vi "Write Body.vi"(8 "error in (no error)":errorcluster, 10 "Body":string="FLATXML", 11 "Annouce Msg in":refnum<class "Annouce Msg.lvclass">) -> (0 "error out":errorcluster, 3 "Annouce Msg out":refnum<class "Annouce Msg.lvclass">)   [LabVIEW 2013, in "Receiver.lvlib" / "Annouce Msg.lvclass"]
uses:
  Annouce Msg.lvclass
  Annouce Msg.lvclass/Annouce Msg.ctl
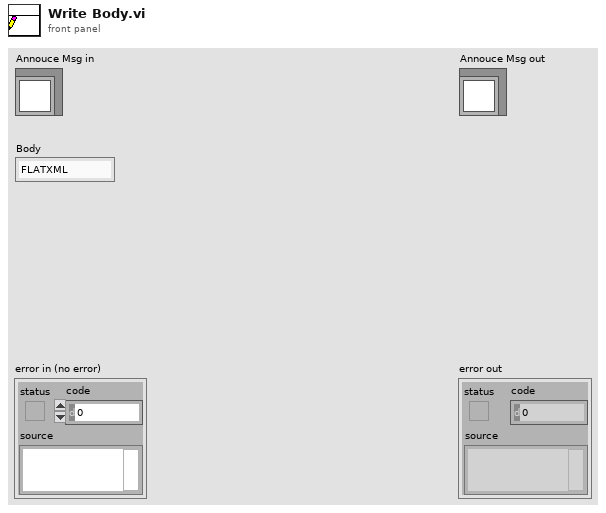
[diagram p1: front panel]
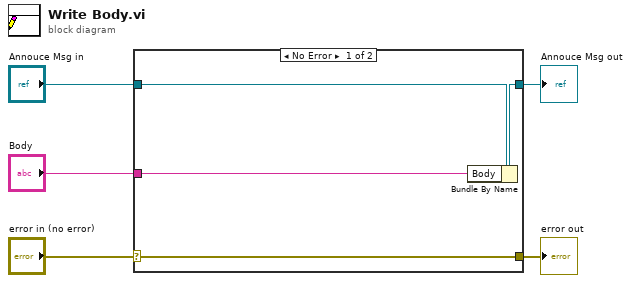
[diagram p0: block diagram]
diagram:
  n1 = case shown="No Error" "error in (no error)" {
    selector: "error in (no error)" -> [w9 w10]
    tunnel: [w9 w10] -> w4
    tunnel: [w7 w11] -> w2
    tunnel: "Annouce Msg in" -> [w8 w11]
    tunnel: "Body" -> [w6 _]
    frame No Error {
      n2 = Bundle By Name(cluster=w8, "Body"=w6) -> (w7:refnum<class "Annouce Msg.lvclass">)
    }
    frame Error {
    }
  }
  "error out" <- w4
  "Annouce Msg out" <- w2
